vi "FPGA AO.vi"() -> ()   [LabVIEW 2017]
uses:
  <vilib>/rvi/Emulation/niFpgaGetClockAttributes.vi
  <vilib>/rvi/Emulation/niFpgaSctlEmulationGetInTimedLoop.vi
  <vilib>/rvi/Emulation/niFpgaEmulationReportErrorSimple.vi
  <vilib>/rvi/eio/common/nirviEmuTemplateMethod_errors.vi
  <vilib>/rvi/Emulation/niFpgaCriticalErrorInLSC.vi
  <vilib>/eio/EIONode/EIONode.xnode
panel:
  out "ConnectorC/AI1":i16
  out "ConnectorC/AI0":i16
  in  "ConnectorC/AO1":i16
  in  "ConnectorC/AO0":i16
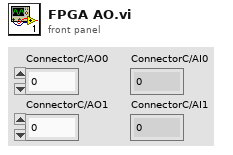
[diagram p1: front panel]
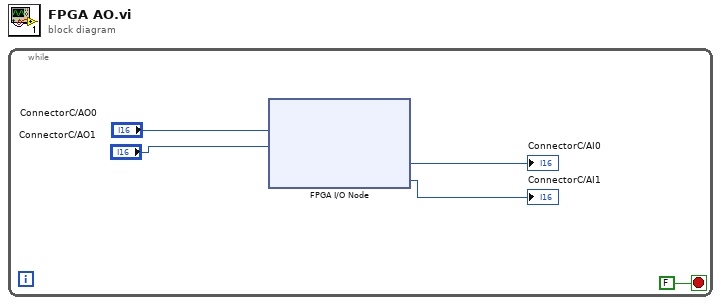
[diagram p0: block diagram]
diagram:
  n1 = while {
    stop <- FALSE stop-if-true
    n2 = xnode "FPGA I/O Node"("ConnectorC/AO0"="ConnectorC/AO0", "ConnectorC/AO1"="ConnectorC/AO1") -> ("ConnectorC/AI0"=→"ConnectorC/AI0":i16, "ConnectorC/AI1"=→"ConnectorC/AI1":i16)  [unwired: 4 in, 4 out]
  }
